vi "Arm Controller.vi"(8 "error in":errorcluster) -> ()   [LabVIEW 2023]
doc: "This VI executes continuously carrying out the current operation and responding to updates or new operations. It will often contain the timing or control code that is difficult to place directly in TeleOp. This VI generally opens all sensors and motors and isolates the rest of the robot code from knowing how the operations are carried out."
uses:
  <vilib>/Rock Robotics/WPI/Framework/Completion Status.ctl
  Arm Setpoints.ctl
  <vilib>/robotics/Kinematics/DH Dynamic Parameters.ctl
  <vilib>/Analysis/Matrix/Datatypes/RealMatrix.ctl
  <vilib>/robotics/Kinematics/DH Kinematic Parameters.ctl
  <vilib>/robotics/Kinematics/Link/Joint Type.ctl
  <vilib>/Rock Robotics/WPI/ThirdParty/REV Robotics/REVLib/Typedef/Spark MAX Control Type.ctl
  <vilib>/Rock Robotics/WPI/Solenoid/WPI_SolenoidValue.ctl
  <vilib>/robotics/Kinematics/Analytical/Initialize Generic Serial Arm.vi
  Framework/Robot Global Data.vi
  <vilib>/Rock Robotics/WPI/Solenoid/WPI_SolenoidSetEnum.vi
  <vilib>/robotics/Kinematics/Robot/Forward Kinematics (Point).vi
  <vilib>/robotics/Kinematics/Generate Cartesian Trajectory (Int).vi
  <vilib>/robotics/Kinematics/Robot/Inverse Kinematics (Point).vi
  <vilib>/robotics/Kinematics/Analytical/NI_Robotics_AnalyticKinematics.lvlib
  <vilib>/Analysis/Matrix/NI_Matrix.lvlib
  <vilib>/robotics/Kinematics/Link/NI_Robotics_Link.lvclass
  <vilib>/robotics/Kinematics/NI_Kinematics.lvlib
  <vilib>/robotics/Kinematics/Robot/NI_Robotics_Serial Robot Arm.lvclass
  <vilib>/Rock Robotics/Network Tables/NT Write Boolean.vi
panel:
  out "Output Lower":dbl
  out "Output Upper":dbl
  out "Sensor Position 4":dbl=277.41477272727275
  out "Sensor Position 3":dbl=225.42613636363637
  out "Applied Output 4":dbl
  out "Applied Output 3":dbl
  out "Applied Output 2":dbl
  in  "Arbitrary Feed Forward (0)":dbl=-0.1
  out "Applied Output":dbl
  out "Sensor Position 6":dbl=331.10795454545456
  out "Sensor Position 5":dbl=278.26704545454544
  in  "PID upper":T1={"P Gain"=0.8, "I Gain"=0.0, "D Gain"=0.0, "F Gain"=0.0, "I Zone"=0.0, "Min Output"=-1.0, "Max Output"=1.0}
  in  "PID Lower":T1={"P Gain"=2.0, "I Gain"=0.0, "D Gain"=0.0, "F Gain"=0.0, "I Zone"=0.0, "Min Output"=-1.0, "Max Output"=1.0}
  out "Sensor Position 2":dbl=187.5
  out "Sensor Position":dbl=124.00568181818183
  out "error out":errorcluster
  in  "Interactive Values":T2
  out "Current\nCmd":string="Started at  12:05:12.296\nDefault: Reserve,  S 0.0, D 0.000000"
  in  "Buttons":cluster{"Execute Cmd":bool, "Abort Cmd":bool}
  out "Command Timing":cluster{"Start Time (ms)":u32, "Iterations":i32}={"Start Time (ms)"=1211869, "Iterations"=0}
  out "Status":T3
  # "Tip: It may be helpful to observe inputs and sensor values.\nYou may also want to display tuning or debugging controls."
  # "Click here to set max"
  # "Click here to set min"
  # "Interactive Command: You may fill in the settings for a command\nand schedule it with the Execute button. You can observe and abort\nany command while fine tuning the code for the controller."
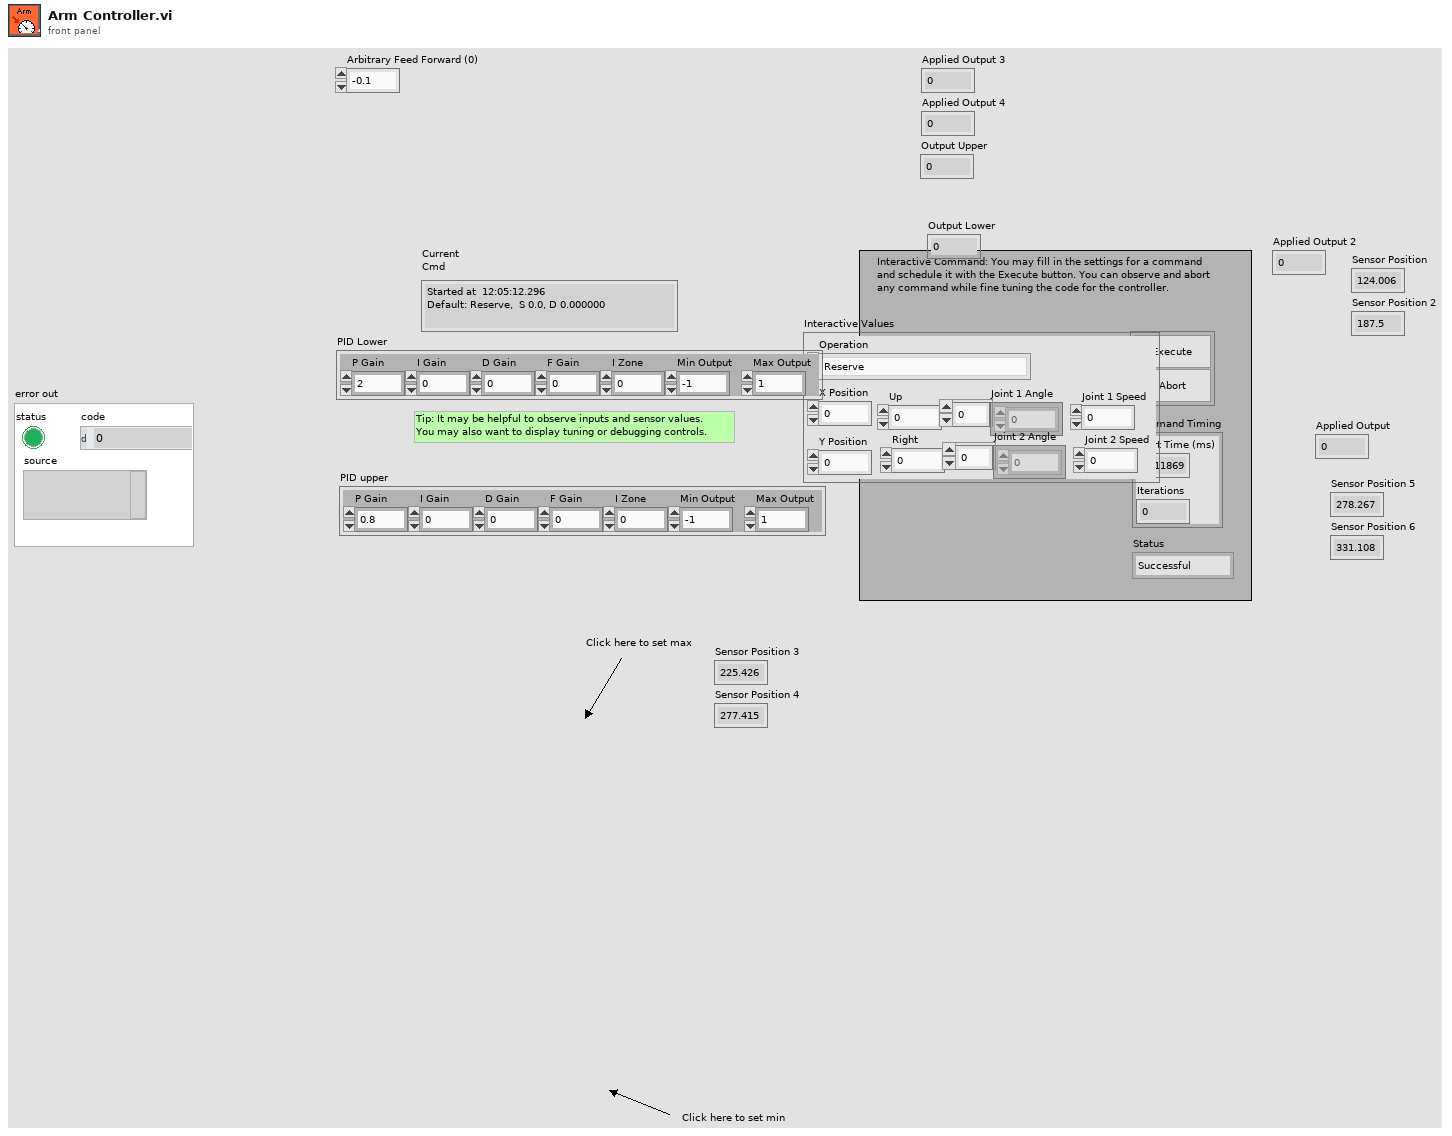
[diagram p1: front panel]
types:
  T1 = cluster{"P Gain":dbl, "I Gain":dbl, "D Gain":dbl, "F Gain":dbl, "I Zone":dbl, "Min Output":dbl, "Max Output":dbl}
  T2 = typedef "Arm Setpoints.ctl" = cluster{"Operation":enum16{"Reserve", "Read Current", "Immediate", "Move to position", "Adjust position", "Cube extend", "Cone extend", "Rotate Arm Joints", "Maintain Angle", "Retract", "Go_to_next"}, "X Position":dbl, "Y Position":dbl, "Up":dbl, "Right":dbl, "Joint 1 Angle":dbl[], "Joint 2 Angle":dbl[], "Joint 1 Speed":dbl, "Joint 2 Speed":dbl}
  T3 = typedef "Completion Status.ctl" = enum16{"Successful", "Aborted", "Incomplete"}
  T4 = typedef "DH Kinematic Parameters.ctl" = cluster{"twist angle":dbl, "length":dbl, "rotation angle":dbl, "offset distance":dbl, "joint type":T5, "joint coordinate offset":dbl}
  T5 = typedef "NI_Robotics_Link.lvclass/Joint Type.ctl" = enum16{"Revolute", "Prismatic"}
  T6 = typedef "DH Dynamic Parameters.ctl" = cluster{"mass":dbl, "gear ratio":dbl, "motor inertia":dbl, "center of gravity":dbl[], "viscous friction":dbl, "positive coulomb friction":dbl, "negative coulomb friction":dbl, "inertia matrix":T7}
  T7 = typedef "NI_Matrix.lvlib/RealMatrix.ctl" = dbl[][]
  T8 = typedef "Command Status Info.ctl" = cluster{"Name":string, "Status":T3, "notifier out":T9}
  T9 = typedef "Completion Notifier.ctl" = refnum<notifier>
  T10 = cluster{"Current Command":T2, "Command Timing":cluster{"Start Time (ms)":u32, "Iterations":i32}, "Command Arguments":cluster{"Command Info":T8, "Description":string, "Default Command":T2, "queue out":refnum<queue>, "Subsystem Name":string}}
  T11 = typedef "Spark MAX Control Type.ctl" = enum16{"Percent VBus", "Voltage", "Velocity", "Position", "Smart Motion", "Current", "Smart Velocity"}
  T12 = typedef "WPI_SolenoidValue.ctl" = enum16{"Off", "On", "Forward", "Reverse"}
  T13 = enum16{"Reserve", "Read Current", "Immediate", "Move to position", "Adjust position", "Cube extend", "Cone extend", "Rotate Arm Joints", "Maintain Angle", "Retract", "Go_to_next"}
  T14 = typedef "WPI_MotorControlDeviceRef.ctl" = cluster{"DeviceStatus":errorcluster, "Type":T15, "PWM":cluster{"PWM Channel":T16, "DeadBand":T17}, "CAN":cluster{"Device Number":u8, "SetOutput VI Ref":variant, "GetOutput VI Ref":variant, "Enable VI Ref":variant, "Disable VI Ref":variant, "Data":variant}, "Invert":bool, "DIO PWM":cluster{"PWM \"Enable\" Channel":T16, "DIOChannel":T18, "PWM Rate":dbl}}
  T15 = typedef "WPI_MotorControlType.ctl" = enum16{"PWM", "CAN", "DIO PWM"}
  T16 = typedef "FPGA_DIOPWMChannel.ctl" = enum8{"PWM 0", "PWM 1", "PWM 2", "PWM 3", "PWM 4", "PWM 5", "PWM 6", "PWM 7", "PWM 8", "PWM 9", "PWM MXP 0", "PWM MXP 1", "PWM MXP 2", "PWM MXP 3", "PWM MXP 4", "PWM MXP 5", "PWM MXP 6", "PWM MXP 7", "PWM MXP 8", "PWM MXP 9", "Invalid"}
  T17 = typedef "WPI_PWMDeadband.ctl" = cluster{"Name":string, "maxPositivePwm":i32, "minPositivePwm":i32, "centerPwm":i32, "maxNegativePwm":i32, "minNegativePwm":i32, "angularRange":u16}
  T18 = typedef "FPGA_DIOChannel.ctl" = enum8{"DIO 0", "DIO 1", "DIO 2", "DIO 3", "DIO 4", "DIO 5", "DIO 6", "DIO 7", "DIO 8", "DIO 9", "DIO MXP 0", "DIO MXP 1", "DIO MXP 2", "DIO MXP 3", "DIO MXP 4", "DIO MXP 5", "DIO MXP 6", "DIO MXP 7", "DIO MXP 8", "DIO MXP 9", "DIO MXP 10", "DIO MXP 11", "DIO MXP 12", "DIO MXP 13", "DIO MXP 14", "DIO MXP 15", "SPI Port CS1", "SPI Port CS2", "SPI Port CS3", "SPI Port MISO", "SPI Port MOSI", "Invalid"}
  T19 = typedef "WPI_SolenoidDevRef.ctl" = cluster{"DevStatus":errorcluster, "Pneumatics Control Module":u8, "Forward Solenoid Channel":T20, "Reverse Solenoid Channel":T20}
  T20 = typedef "WPI_SolenoidChannel.ctl" = enum8{"Solenoid 0", "Solenoid 1", "Solenoid 2", "Solenoid 3", "Solenoid 4", "Solenoid 5", "Solenoid 6", "Solenoid 7", "Solenoid 8", "Solenoid 9", "Solenoid 10", "Solenoid 11", "Solenoid 12", "Solenoid 13", "Solenoid 14", "Solenoid 15", "Invalid"}
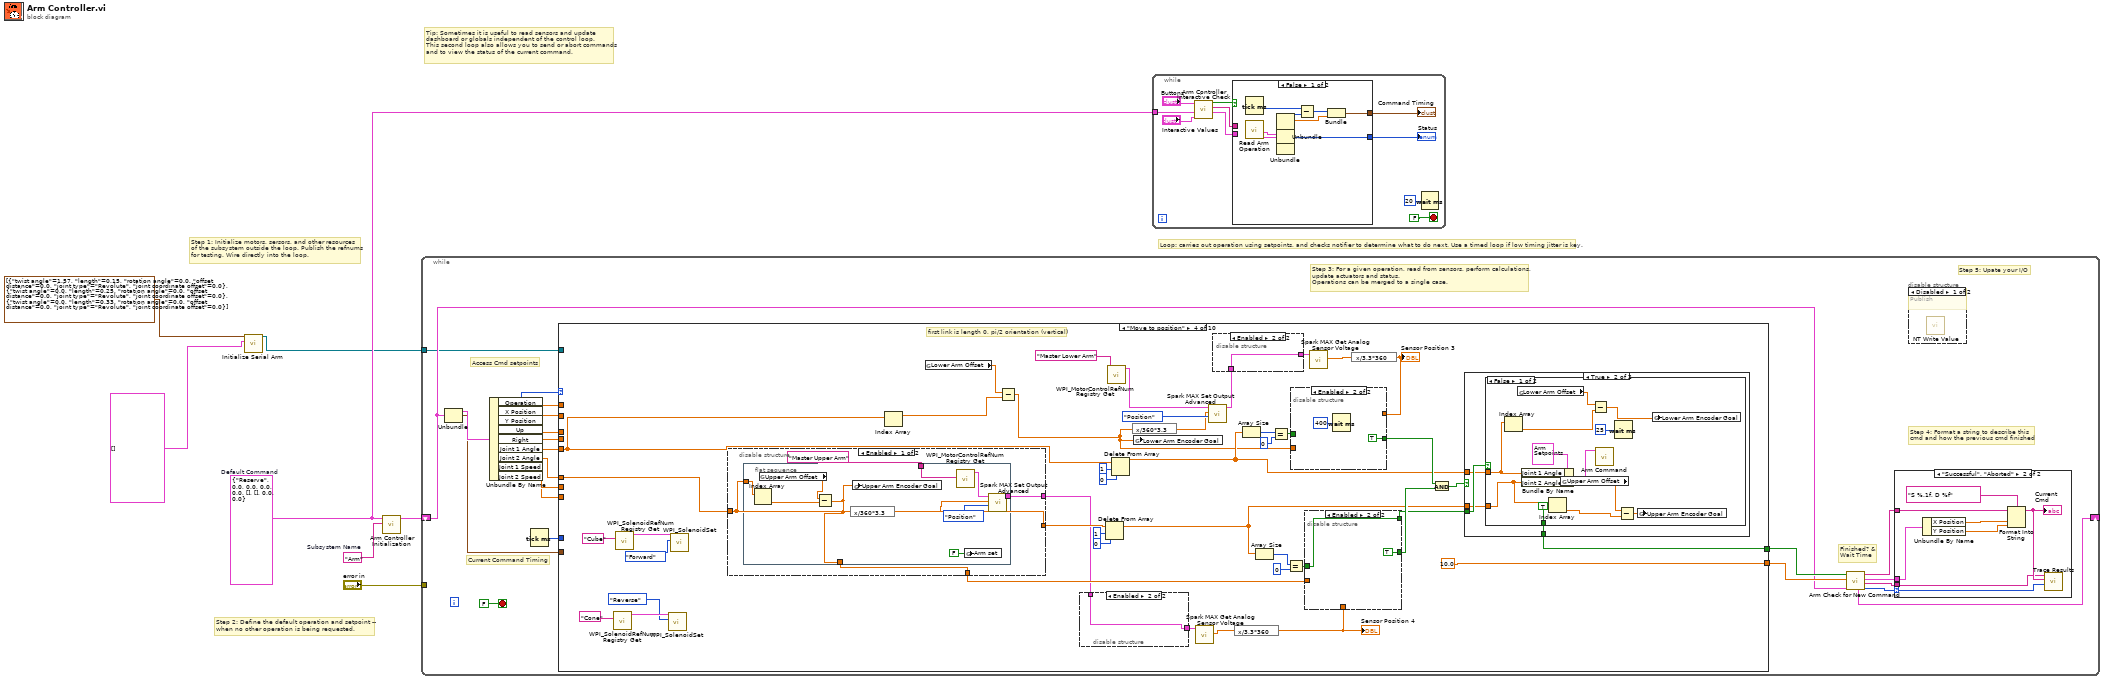
[diagram p0: block diagram]
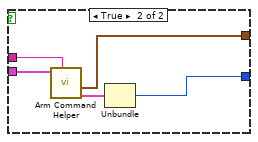
[diagram p2: hidden frame]
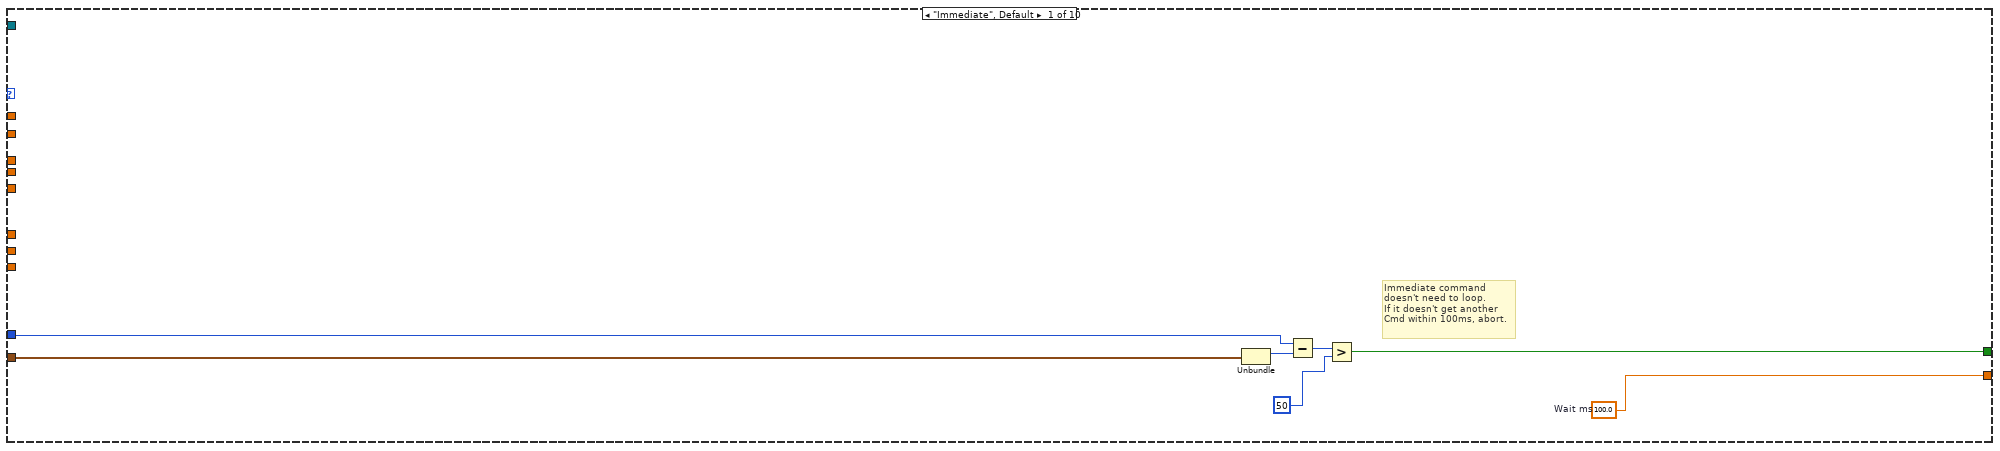
[diagram p3: hidden frame]
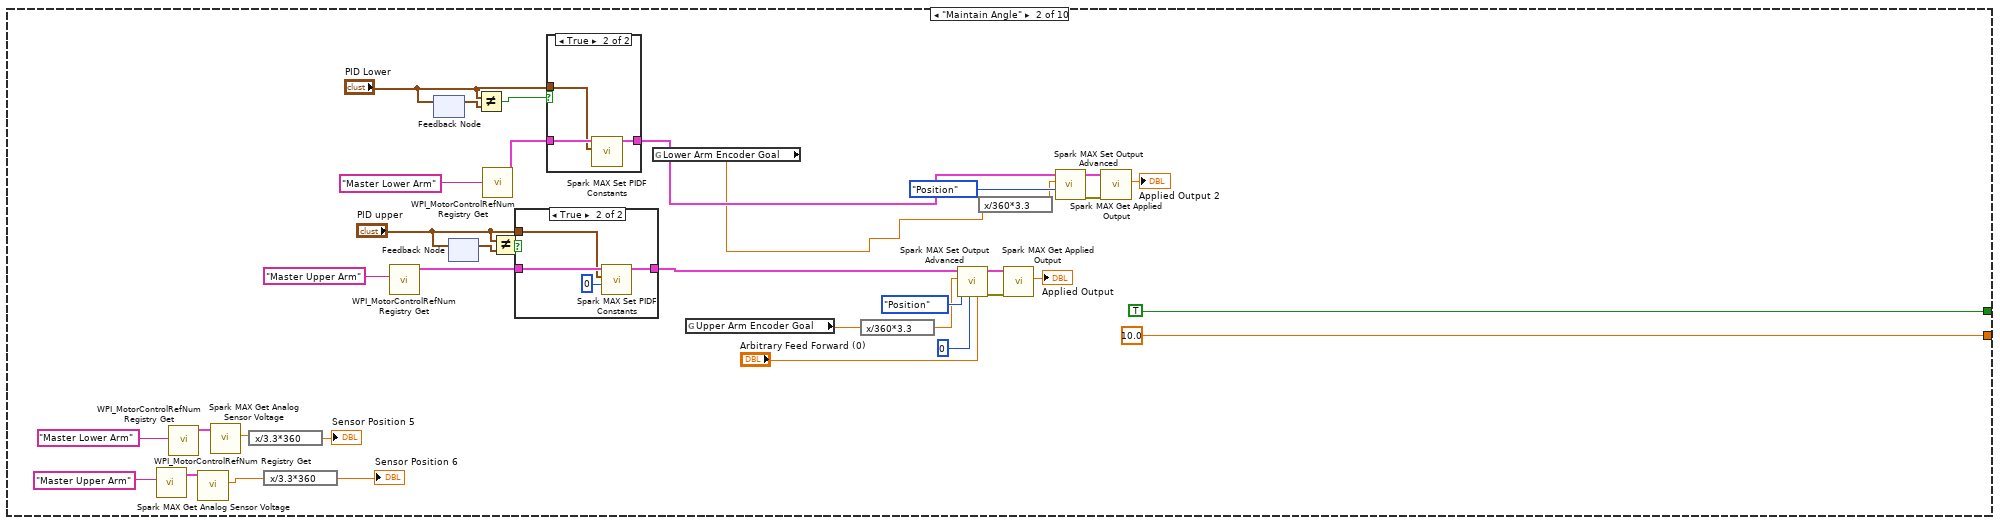
[diagram p4: hidden frame]
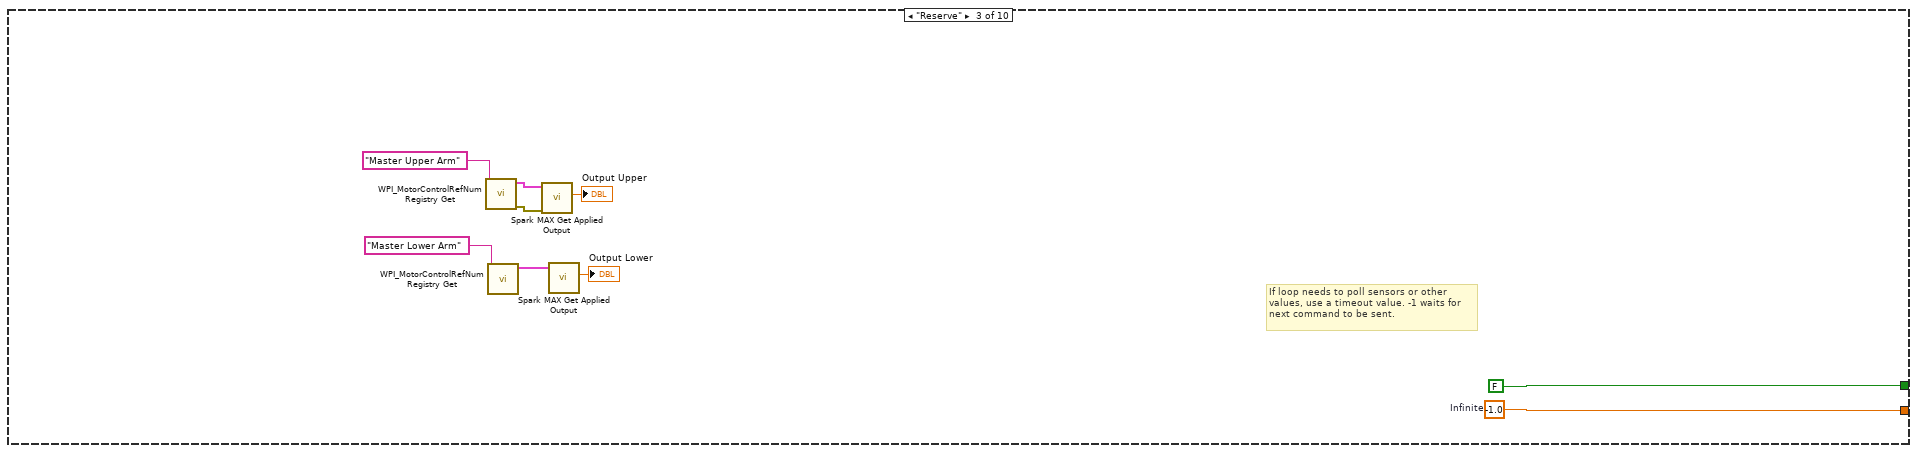
[diagram p7: hidden frame]
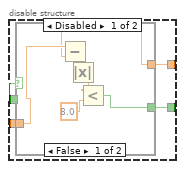
[diagram p8: hidden frame]
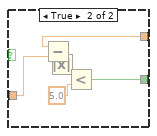
[diagram p9: hidden frame]
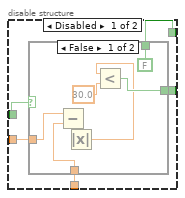
[diagram p10: hidden frame]
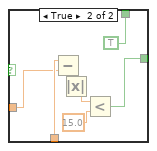
[diagram p11: hidden frame]
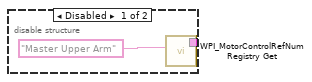
[diagram p12: hidden frame]
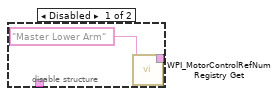
[diagram p13: hidden frame]
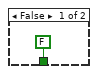
[diagram p14: hidden frame]
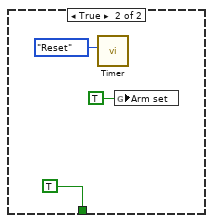
[diagram p15: hidden frame]
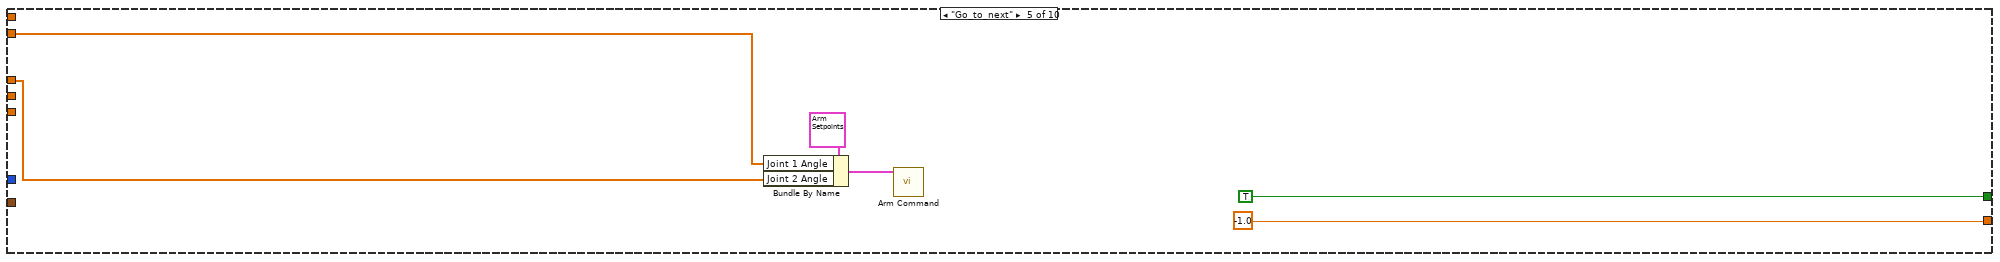
[diagram p17: hidden frame]
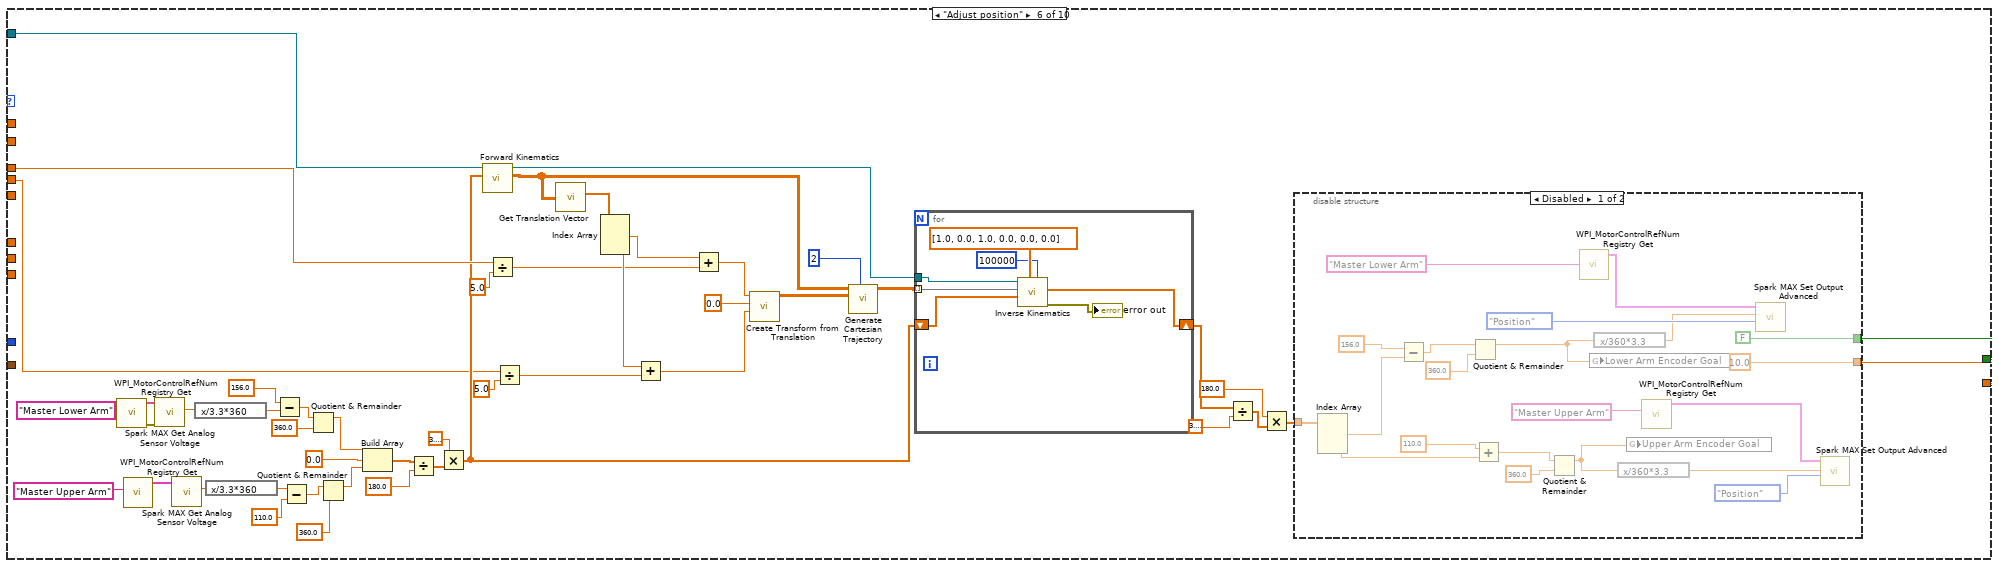
[diagram p18: hidden frame]
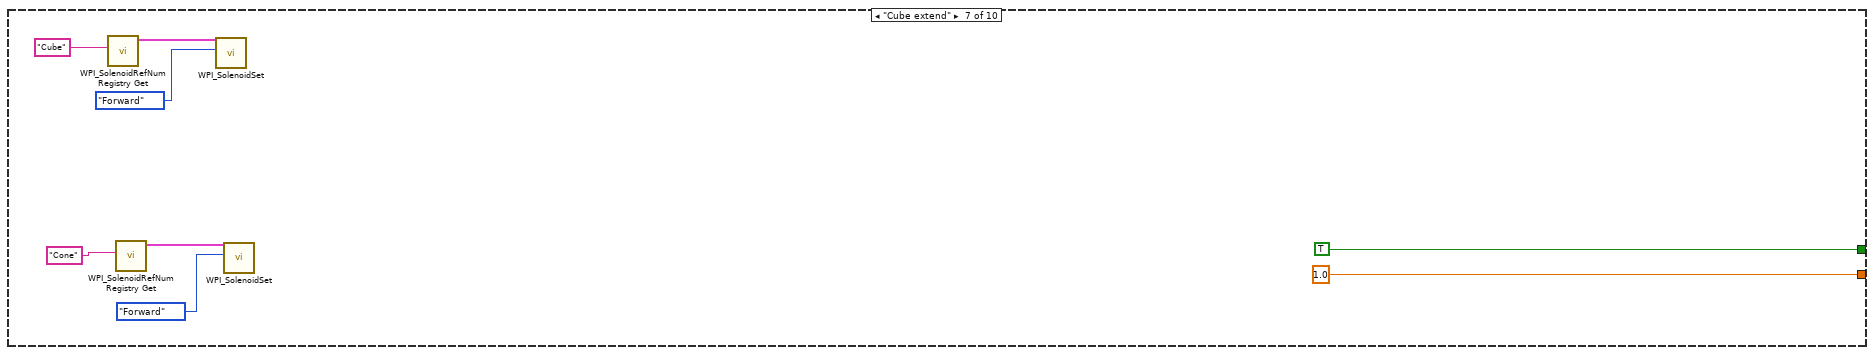
[diagram p20: hidden frame]
diagram:
  w4 = T2 {"Operation"=enum."Reserve", "X Position"=0.0, "Y Position"=0.0, "Up"=0.0, "Right"=0.0, "Joint 1 Angle"=[], "Joint 2 Angle"=[], "Joint 1 Speed"=0.0, "Joint 2 Speed"=0.0}  # Default Command
  w5 = "Arm"  # Subsystem Name
  # "Tip: Sometimes it is useful to read sensors and update\ndashboard or globals independent of the control loop.\nThis second loop also allows you to send or abort commands\nand to view the status of the current command."
  # "Step 2: Define the default operation and setpoint --\nwhen no other operation is being requested."
  # "Step 1: Initialize motors, sersors, and other resources\nof the subsystem outside the loop. Publish the refnums\nfor testing. Wire directly into the loop."
  # "Loop: carries out operation using setpoints, and checks notifier to determine what to do next. Use a timed loop if low timing jitter is key."
  n1 = call-poly <vilib>:"Initialize Serial Arm.vi"("dynamic parameters"=T6[] [], "kinematic parameters"=T4[] [{"twist angle"=1.57, "length"=0.15, "rotation angle"=0.0, "offset distance"=0.0, "joint type"=enum."Revolute", "joint coordinate offset"=0.0}, {"twist angle"=0.0, "length"=0.25, "rotation angle"=0.0, "offset distance"=0.0, "joint type"=enum."Revolute", "joint coordinate offset"=0.0}, {"twist angle"=0.0, "length"=0.33, "rotation angle"=0.0, "offset distance"=0.0, "joint type"=enum."Revolute", "joint coordinate offset"=0.0}]) -> ("serial arm out"=w1:refnum<class "NI_Robotics_Serial Robot Arm.lvclass">)  [unwired: 8 in, 1 out]
  n2 = call "Arm Controller Initialization.vi"("Subsystem Name"=w5, "Default Command"=w4) -> ("Current Command"=w6:T10)  [unwired: 9 in]
  n3 = while {
    shift-right: [w22] -> _
    shift-left: w6 -> [w15]
    tunnel: "error in" -> [_]
    tunnel: w1 -> [w14]
    stop <- FALSE stop-if-true
    # "Step 5: Upate your I/O"
    # "Step 4: Format a string to describe this\ncmd and how the previous cmd finished"
    # "Current Command Timing"
    # "Access Cmd setpoints"
    # "Finished? &\nWait Time"
    # "Step 3: For a given operation, read from sensors, perform calculations,\nupdate actuators and status.\nOperations can be merged to a single case."
    n4 = Unbundle(w15) -> ("Current Command"=w28:T2, "Command Timing"=w24:cluster{"Start Time (ms)":u32, "Iterations":i32})  [unwired: 1 out]
    n5 = Unbundle By Name(w28) -> ("Operation"=w27:T13, "X Position"=w26:dbl, "Y Position"=w23:dbl, "Up"=w13:dbl, "Right"=w12:dbl, "Joint 1 Angle"=w11:dbl[], "Joint 2 Angle"=w10:dbl[], "Joint 1 Speed"=w9:dbl, "Joint 2 Speed"=w8:dbl)
    n6 = Tick Count (ms)() -> (millisecond timer value=w25:u32)
    n7 = case shown="\"Move to position\"" w27 {
      tunnel: [w36 10.0 ("Infinite") w90 10.0 ("Infinite") -1.0 ("Infinite") w250 1.0 ("Infinite") 1.0 ("Infinite") 1.0 ("Infinite") 100.0 ("Infinite")] -> w20
      tunnel: [w30 TRUE ("ignore previous (F)") FALSE ("ignore previous (F)") w112 TRUE ("ignore previous (F)") w251 TRUE ("ignore previous (F)") TRUE ("ignore previous (F)") TRUE ("ignore previous (F)") TRUE ("ignore previous (F)")] -> w21
      tunnel: w24 -> [w32 _ _ _ _ _ _ _ _ _]
      tunnel: w26 -> [_ _ _ _ _ _ _ _ _ _]
      tunnel: w25 -> [w31 _ _ _ _ _ _ _ _ _]
      tunnel: w23 -> [_ _ _ _ _ _ _ _ _ _]
      tunnel: w14 -> [_ _ _ _ _ w258 _ _ _ _]
      tunnel: w13 -> [_ _ _ _ _ w252 _ _ _ _]
      tunnel: w12 -> [_ _ _ _ _ w236 _ _ _ _]
      tunnel: w11 -> [_ _ _ w102 w216 _ _ _ _ _]
      tunnel: w10 -> [_ _ _ w103 w215 _ _ _ _ _]
      tunnel: w9 -> [_ _ _ _ _ _ _ _ _ w341]
      tunnel: w8 -> [_ _ _ _ _ _ _ _ _ w340]
      frame "Immediate", Default {
        w36 = 100.0  # Wait ms
        # "Immediate command\ndoesn't need to loop.\nIf it doesn't get another\nCmd within 100ms, abort."
        n8 = Unbundle(w32) -> ("Start Time (ms)"=w35:u32)  [unwired: 1 out]
        n9 = Subtract(x=w31, y=w35) -> (x-y=w34:u32)
        n10 = Greater?(x=w34, y=u8 50 ("Left Motor")) -> (0:w30:bool)
      }
      frame "Maintain Angle" {
        n11 = call <vilib>:"WPI_MotorControlRefNum Registry Get.vi"("refnum name"="Master Upper Arm") -> ("MotorControlDevRef"=w59:T14)  [unwired: 9 in, 1 out]
        n12 = call <vilib>:"WPI_MotorControlRefNum Registry Get.vi"("refnum name"="Master Lower Arm") -> ("MotorControlDevRef"=w60:T14)  [unwired: 9 in, 1 out]
        n13 = call <vilib>:"Spark MAX Get Analog Sensor Voltage.vi"("MotorControlDevRef in"=w59) -> ("Analog Sensor Voltage"=w58:dbl)  [unwired: 7 in, 3 out]
        n14 = call <vilib>:"Spark MAX Get Analog Sensor Voltage.vi"("MotorControlDevRef in"=w60) -> ("Analog Sensor Voltage"=w57:dbl)  [unwired: 7 in, 3 out]
        n15 = expression code="x/3.3*360"(w57) -> (→"Sensor Position 5":dbl)
        n16 = expression code="x/3.3*360"(w58) -> (→"Sensor Position 6":dbl)
        n17 = call <vilib>:"WPI_MotorControlRefNum Registry Get.vi"("refnum name"="Master Upper Arm") -> ("MotorControlDevRef"=w69:T14)  [unwired: 9 in, 1 out]
        n18 = feedback #1() -> (w53:T1)  [unwired: 1 in]
        n19 = feedback-in #1("PID Lower") -> ()
        n20 = feedback-in #2("PID upper") -> ()
        n21 = feedback #2() -> (w55:T1)  [unwired: 1 in]
        n22 = Not Equal?(x="PID Lower", y=w53) -> (x != y?=w52:bool)
        n23 = call <vilib>:"WPI_MotorControlRefNum Registry Get.vi"("refnum name"="Master Lower Arm") -> ("MotorControlDevRef"=w71:T14)  [unwired: 9 in, 1 out]
        n24 = Not Equal?(x="PID upper", y=w55) -> (x != y?=w54:bool)
        n25 = case shown="True" w54 {
          tunnel: w69 -> [w77 w81]
          tunnel: "PID upper" -> [_ w80]
          tunnel: [w77 w79] -> w67
          frame False {
          }
          frame True {
            n26 = call <vilib>:"Spark MAX Set PIDF Constants.vi"("PIDF Slot"=0, "PID Constants"=w80, "MotorControlDeviceRef"=w81) -> ("MotorControlDeviceRef"=w79:T14)  [unwired: 7 in, 1 out]
          }
        }
        n27 = case shown="True" w52 {
          tunnel: w71 -> [w73 w76]
          tunnel: [w73 w75] -> w68
          tunnel: "PID Lower" -> [_ w74]
          frame False {
          }
          frame True {
            n28 = call <vilib>:"Spark MAX Set PIDF Constants.vi"("PID Constants"=w74, "MotorControlDeviceRef"=w76) -> ("MotorControlDeviceRef"=w75:T14)  [unwired: 8 in, 1 out]
          }
        }
        n29 = global read "Robot Global Data.vi" "Lower Arm Encoder Goal"() -> (w38:dbl)
        n30 = global read "Robot Global Data.vi" "Upper Arm Encoder Goal"() -> (w37:dbl)
        n31 = expression code="x/360*3.3"(w37) -> (w44:dbl)
        n32 = call <vilib>:"Spark MAX Set Output Advanced.vi"("Arbitrary Feed Forward (0)"="Arbitrary Feed Forward (0)", "PIDF Slot (0)"=0, "Control Mode"=Spark_MAX_Control_Type."Position", "Setpoint"=w44, "MotorControlDevRef"=w67) -> ("error out"=w49:errorcluster, "MotorControlDevRef"=w48:T14)  [unwired: 5 in]
        n33 = expression code="x/360*3.3"(w38) -> (w42:dbl)
        n34 = call <vilib>:"Spark MAX Get Applied Output.vi"("error in (no error)"=w49, "MotorControlDevRef in"=w48) -> ("Applied Output"=→"Applied Output":dbl)  [unwired: 6 in, 3 out]
        n35 = call <vilib>:"Spark MAX Set Output Advanced.vi"("Control Mode"=Spark_MAX_Control_Type."Position", "Setpoint"=w42, "MotorControlDevRef"=w68) -> ("error out"=w39:errorcluster, "MotorControlDevRef"=w40:T14)  [unwired: 7 in]
        n36 = call <vilib>:"Spark MAX Get Applied Output.vi"("error in (no error)"=w39, "MotorControlDevRef in"=w40) -> ("Applied Output"=→"Applied Output 2":dbl)  [unwired: 6 in, 3 out]
      }
      frame "Reserve" {
        w90 = -1.0  # Infinite
        # "If loop needs to poll sensors or other\nvalues, use a timeout value. -1 waits for\nnext command to be sent."
        n37 = call <vilib>:"WPI_MotorControlRefNum Registry Get.vi"("refnum name"="Master Upper Arm") -> ("error out"=w86:errorcluster, "MotorControlDevRef"=w85:T14)  [unwired: 9 in]
        n38 = call <vilib>:"WPI_MotorControlRefNum Registry Get.vi"("refnum name"="Master Lower Arm") -> ("MotorControlDevRef"=w82:T14)  [unwired: 9 in, 1 out]
        n39 = call <vilib>:"Spark MAX Get Applied Output.vi"("error in (no error)"=w86, "MotorControlDevRef in"=w85) -> ("Applied Output"=→"Output Upper":dbl)  [unwired: 6 in, 3 out]
        n40 = call <vilib>:"Spark MAX Get Applied Output.vi"("MotorControlDevRef in"=w82) -> ("Applied Output"=→"Output Lower":dbl)  [unwired: 7 in, 3 out]
      }
      frame "Move to position" {
        # "first link is length 0, pi/2 orientation (vertical)"
        n41 = call <vilib>:"WPI_SolenoidRefNum Registry Get.vi"("refnum name"="Cone") -> ("SolenoidDevRef"=w106:T19)  [unwired: 9 in, 1 out]
        n42 = call <vilib>:"WPI_SolenoidRefNum Registry Get.vi"("refnum name"="Cube") -> ("SolenoidDevRef"=w109:T19)  [unwired: 9 in, 1 out]
        n43 = call-poly <vilib>:"WPI_SolenoidSet.vi"("Value"=WPI_SolenoidValue."Reverse", "SolenoidDevRef"=w106) -> ()  [unwired: 8 in, 2 out]
        n44 = call-poly <vilib>:"WPI_SolenoidSet.vi"("Value"=WPI_SolenoidValue."Forward", "SolenoidDevRef"=w109) -> ()  [unwired: 8 in, 2 out]
        n45 = disable-structure shown="Enabled" {
          disable-tunnel: w103 -> [w201 _]
          disable-tunnel: [w201 _] -> w125
          disable-tunnel: [w200 _] -> w115
          disable-tunnel: [w199 _] -> w97
          frame Enabled {
            n46 = flat-sequence {
              tunnel: "Master Upper Arm" ("refnum name") -> [w210]
              tunnel: w201 -> [w209]
              tunnel: [w205] -> w200
              tunnel: [w206] -> w199
              frame #0 {
                n47 = Index Array(array=w209) -> (element=w203:dbl)  [unwired: 1 in]
                n48 = global read "Robot Global Data.vi" "Upper Arm Offset"() -> (w204:dbl)
                n49 = Subtract(x=w204, y=w203) -> (x-y=w205:dbl)
                n50 = expression code="x/360*3.3"(w205) -> (w208:dbl)
                n51 = global write "Robot Global Data.vi" "Upper Arm Encoder Goal"(w205) -> ()
                n52 = call <vilib>:"WPI_MotorControlRefNum Registry Get.vi"("refnum name"=w210) -> ("MotorControlDevRef"=w211:T14)  [unwired: 9 in, 1 out]
                n53 = global write "Robot Global Data.vi" "Arm set"(FALSE ("Arm set")) -> ()
                n54 = call <vilib>:"Spark MAX Set Output Advanced.vi"("Control Mode"=Spark_MAX_Control_Type."Position", "Setpoint"=w208, "MotorControlDevRef"=w211) -> ("MotorControlDevRef"=w206:T14)  [unwired: 7 in, 1 out]
              }
            }
          }
          frame Disabled {
          }
        }
        n55 = Index Array(array=w102) -> (element=w91:dbl)  [unwired: 1 in]
        n56 = global read "Robot Global Data.vi" "Lower Arm Offset"() -> (w92:dbl)
        n57 = Subtract(x=w92, y=w91) -> (x-y=w93:dbl)
        n58 = disable-structure shown="Enabled" {
          disable-tunnel: [w173 w175] -> w119
          disable-tunnel: w97 -> [_ w175]
          frame Disabled {
            n59 = call <vilib>:"WPI_MotorControlRefNum Registry Get.vi"("refnum name"="Master Upper Arm") -> ("MotorControlDevRef"=w173:T14)  [unwired: 9 in, 1 out]
          }
          frame Enabled {
          }
        }
        n60 = Delete From Array(array=w125, length=1, index=0) -> (array with subset deleted=w110:dbl[])  [unwired: 1 out]
        n61 = call <vilib>:"WPI_MotorControlRefNum Registry Get.vi"("refnum name"="Master Lower Arm") -> ("MotorControlDevRef"=w130:T14)  [unwired: 9 in, 1 out]
        n62 = Delete From Array(array=w102, length=1, index=0) -> (array with subset deleted=w111:dbl[])  [unwired: 1 out]
        n63 = expression code="x/360*3.3"(w93) -> (w101:dbl)
        n64 = global write "Robot Global Data.vi" "Lower Arm Encoder Goal"(w93) -> ()
        n65 = call <vilib>:"Spark MAX Get Analog Sensor Voltage.vi"("MotorControlDevRef in"=w119) -> ("Analog Sensor Voltage"=w118:dbl)  [unwired: 7 in, 3 out]
        n66 = call <vilib>:"Spark MAX Set Output Advanced.vi"("Control Mode"=Spark_MAX_Control_Type."Position", "Setpoint"=w101, "MotorControlDevRef"=w130) -> ("MotorControlDevRef"=w98:T14)  [unwired: 7 in, 1 out]
        n67 = disable-structure shown="Enabled" {
          disable-tunnel: [w176 w178] -> w120
          disable-tunnel: w98 -> [_ w178]
          frame Disabled {
            n68 = call <vilib>:"WPI_MotorControlRefNum Registry Get.vi"("refnum name"="Master Lower Arm") -> ("MotorControlDevRef"=w176:T14)  [unwired: 9 in, 1 out]
          }
          frame Enabled {
          }
        }
        n69 = expression code="x/3.3*360"(w118) -> (w99:dbl)
        "Sensor Position 4" <- w99
        n70 = Array Size(array=w111) -> (size(s)=w122:i32)
        n71 = Array Size(array=w110) -> (size(s)=w95:i32)
        n72 = Equal?(x=w122, y=0) -> (x = y?=w123:bool)
        n73 = Equal?(x=w95, y=0) -> (x = y?=w96:bool)
        n74 = disable-structure shown="Enabled" {
          disable-tunnel: w115 -> [w156 _]
          disable-tunnel: [w155 TRUE] -> w114
          disable-tunnel: [w154 w171] -> w113
          disable-tunnel: w99 -> [w153 _]
          disable-tunnel: w96 -> [w152 w171]
          frame Disabled {
            n75 = case shown="False" w152 {
              tunnel: w156 -> [w159 w164]
              tunnel: [w162 w169] -> w155
              tunnel: [FALSE TRUE] -> w154
              tunnel: w153 -> [w158 w166]
              frame False {
                n76 = Subtract(x=w159, y=w158) -> (x-y=w160:dbl)
                n77 = Absolute Value(x=w160) -> (abs(x)=w157:dbl)
                n78 = Less?(x=w157, y=30.0) -> (x < y?=w162:bool)
              }
              frame True {
                n79 = Subtract(x=w166, y=w164) -> (x-y=w167:dbl)
                n80 = Absolute Value(x=w167) -> (abs(x)=w165:dbl)
                n81 = Less?(x=w165, y=15.0) -> (x < y?=w169:bool)
              }
            }
          }
          frame Enabled {
          }
        }
        n82 = call <vilib>:"Spark MAX Get Analog Sensor Voltage.vi"("MotorControlDevRef in"=w120) -> ("Analog Sensor Voltage"=w117:dbl)  [unwired: 7 in, 3 out]
        n83 = expression code="x/3.3*360"(w117) -> (w100:dbl)
        "Sensor Position 3" <- w100
        n84 = disable-structure shown="Enabled" {
          disable-tunnel: w123 -> [w137 _]
          disable-tunnel: [w136 TRUE] -> w116
          disable-tunnel: w93 -> [w135 _]
          disable-tunnel: w100 -> [w134 _]
          frame Disabled {
            n85 = case shown="False" w137 {
              tunnel: [w142 w149] -> w136
              tunnel: w135 -> [w139 w146]
              tunnel: w134 -> [w138 w144]
              frame False {
                n86 = Subtract(x=w139, y=w138) -> (x-y=w141:dbl)
                n87 = Absolute Value(x=w141) -> (abs(x)=w140:dbl)
                n88 = Less?(x=w140, y=8.0) -> (x < y?=w142:bool)
              }
              frame True {
                n89 = Subtract(x=w144, y=w146) -> (x-y=w147:dbl)
                n90 = Absolute Value(x=w147) -> (abs(x)=w145:dbl)
                n91 = Less?(x=w145, y=5.0) -> (x < y?=w149:bool)
              }
            }
          }
          frame Enabled {
            n92 = Wait (ms)(milliseconds to wait=u32 400) -> ()  [unwired: 1 out]
          }
        }
        n93 = And(x=w116, y=w114) -> (x .and. y?=w121:bool)
        n94 = case shown="True" w121 {
          tunnel: w113 -> [_ w183]
          tunnel: [FALSE w182] -> w112
          tunnel: w111 -> [_ w181]
          tunnel: w110 -> [_ w180]
          frame False {
          }
          frame True {
            n95 = case shown="False" w183 {
              tunnel: [TRUE TRUE] -> w182
              tunnel: w181 -> [w191 _]
              tunnel: w180 -> [w190 _]
              frame False {
                n96 = Index Array(array=w191) -> (element=w185:dbl)  [unwired: 1 in]
                n97 = global read "Robot Global Data.vi" "Lower Arm Offset"() -> (w186:dbl)
                n98 = Bundle By Name(cluster=T2 {"Operation"=enum."Move to position", "X Position"=0.0, "Y Position"=0.0, "Up"=0.0, "Right"=0.0, "Joint 1 Angle"=[], "Joint 2 Angle"=[], "Joint 1 Speed"=0.0, "Joint 2 Speed"=0.0} ("SubSystem Data"), "Joint 1 Angle"=w191, "Joint 2 Angle"=w190) -> (w193:T2)
                n99 = Index Array(array=w190) -> (element=w188:dbl)  [unwired: 1 in]
                n100 = global read "Robot Global Data.vi" "Upper Arm Offset"() -> (w189:dbl)
                n101 = Subtract(x=w186, y=w185) -> (x-y=w184:dbl)
                n102 = call "Arm Command.vi"("SubSystem Data"=w193) -> ()  [unwired: 10 in, 1 out]
                n103 = Wait (ms)(milliseconds to wait=u32 25 ("millisecond timer value")) -> ()  [unwired: 1 out]
                n104 = Subtract(x=w189, y=w188) -> (x-y=w187:dbl)
                n105 = global write "Robot Global Data.vi" "Upper Arm Encoder Goal"(w187) -> ()
                n106 = global write "Robot Global Data.vi" "Lower Arm Encoder Goal"(w184) -> ()
              }
              frame True {
                n107 = call "Timer.vi"("Action"=enum16{"Reset", "Get"}."Reset") -> ()  [unwired: 10 in, 1 out]
                n108 = global write "Robot Global Data.vi" "Arm set"(TRUE ("Arm set")) -> ()
              }
            }
          }
        }
      }
      frame "Go_to_next" {
        n109 = Bundle By Name(cluster=T2 {"Operation"=enum."Move to position", "X Position"=0.0, "Y Position"=0.0, "Up"=0.0, "Right"=0.0, "Joint 1 Angle"=[], "Joint 2 Angle"=[], "Joint 1 Speed"=0.0, "Joint 2 Speed"=0.0} ("SubSystem Data"), "Joint 1 Angle"=w216, "Joint 2 Angle"=w215) -> (w217:T2)
        n110 = call "Arm Command.vi"("SubSystem Data"=w217) -> ()  [unwired: 10 in, 1 out]
      }
      frame "Adjust position" {
        n111 = call <vilib>:"WPI_MotorControlRefNum Registry Get.vi"("refnum name"="Master Lower Arm") -> ("error out"=w232:errorcluster, "MotorControlDevRef"=w233:T14)  [unwired: 9 in]
        n112 = call <vilib>:"WPI_MotorControlRefNum Registry Get.vi"("refnum name"="Master Upper Arm") -> ("MotorControlDevRef"=w230:T14)  [unwired: 9 in, 1 out]
        n113 = call <vilib>:"Spark MAX Get Analog Sensor Voltage.vi"("error in (no error)"=w232, "MotorControlDevRef in"=w233) -> ("Analog Sensor Voltage"=w231:dbl)  [unwired: 6 in, 3 out]
        n114 = call <vilib>:"Spark MAX Get Analog Sensor Voltage.vi"("MotorControlDevRef in"=w230) -> ("Analog Sensor Voltage"=w229:dbl)  [unwired: 7 in, 3 out]
        n115 = expression code="x/3.3*360"(w231) -> (w228:dbl)
        n116 = expression code="x/3.3*360"(w229) -> (w223:dbl)
        n117 = Subtract(x=156.0, y=w228) -> (x-y=w225:dbl)
        n118 = Subtract(x=w223, y=110.0) -> (x-y=w221:dbl)
        n119 = Quotient & Remainder(x=w225, y=360.0) -> (x-y*floor(x/y)=w226:dbl)  [unwired: 1 out]
        n120 = Quotient & Remainder(x=w221, y=360.0) -> (x-y*floor(x/y)=w219:dbl)  [unwired: 1 out]
        n121 = Build Array(w226, 0.0 ("element"), w219) -> (w247:dbl[])
        n122 = Divide(x=w247, y=180.0 ("x")) -> (x/y=w266:dbl[])
        n123 = Multiply(x=3.141592653589793, y=w266) -> (x*y=w245:dbl[])
        n124 = call-poly <vilib>:"Forward Kinematics.vi"("joint positions"=w245, "serial arm in"=w258) -> ("end effector transform"=w243:T7, "serial arm out"=w261:refnum<class "NI_Robotics_Serial Robot Arm.lvclass">)  [unwired: 7 in, 1 out]
        n125 = Divide(x=w252, y=5.0) -> (x/y=w238:dbl)
        n126 = Divide(x=w236, y=5.0) -> (x/y=w235:dbl)
        n127 = call <vilib>:"Get Translation Vector.vi"("transform"=w243) -> ("translation vector"=w242:dbl[])
        n128 = Index Array(array=w242) -> (element #1=w241:dbl, element #3=w240:dbl)  [unwired: 3 in, 1 out]
        n129 = Add(x=w240, y=w235) -> (x+y=w253:dbl)
        n130 = Add(x=w241, y=w238) -> (x+y=w244:dbl)
        n131 = call <vilib>:"Create Transform from Translation.vi"("z"=w253, "y"=0.0, "x"=w244) -> ("transform"=w262:T7)  [unwired: 8 in]
        n132 = call-poly <vilib>:"Generate Cartesian Trajectory.vi"("intermediate points"=2, "end transform"=w262, "start transform"=w243) -> ("interpolated trajectory"=w260:dbl[][][])  [unwired: 7 in, 1 out]
        n133 = for {
          tunnel: w261 -> [w294]
          tunnel: w260 -> [w293] mode=indexing
          shift-right: [w288] -> w254
          shift-left: w245 -> [w289]
          n134 = call-poly <vilib>:"Inverse Kinematics.vi"("max steps"=100000, "mask"=dbl[] [1.0, 0.0, 1.0, 0.0, 0.0, 0.0], "current joint positions"=w289, "end effector transform"=w293, "serial arm in"=w294) -> ("error out"=→"error out":errorcluster, "joint positions"=w288:dbl[])  [unwired: 3 in, 2 out]
        }
        n135 = Divide(x=w254, y=3.141592653589793) -> (x/y=w255:dbl[])
        n136 = Multiply(x=180.0, y=w255) -> (x*y=w248:dbl[])
        n137 = disable-structure shown="Disabled" {
          disable-tunnel: [FALSE ("ignore previous (F)") _] -> w251
          disable-tunnel: [10.0 ("Infinite") _] -> w250
          disable-tunnel: w248 -> [w285 _]
          frame Disabled {
            n138 = Index Array(array=w285) -> (element #1=w276:dbl, element #3=w273:dbl)  [unwired: 3 in, 1 out]
            n139 = Subtract(x=156.0, y=w276) -> (x-y=w271:dbl)
            n140 = Quotient & Remainder(x=w271, y=360.0) -> (x-y*floor(x/y)=w270:dbl)  [unwired: 1 out]
            n141 = Add(x=110.0, y=w273) -> (x+y=w268:dbl)
            n142 = Quotient & Remainder(x=w268, y=360.0) -> (x-y*floor(x/y)=w267:dbl)  [unwired: 1 out]
            n143 = call <vilib>:"WPI_MotorControlRefNum Registry Get.vi"("refnum name"="Master Lower Arm") -> ("MotorControlDevRef"=w279:T14)  [unwired: 9 in, 1 out]
            n144 = global write "Robot Global Data.vi" "Lower Arm Encoder Goal"(w270) -> ()
            n145 = expression code="x/360*3.3"(w270) -> (w281:dbl)
            n146 = expression code="x/360*3.3"(w267) -> (w283:dbl)
            n147 = global write "Robot Global Data.vi" "Upper Arm Encoder Goal"(w267) -> ()
            n148 = call <vilib>:"WPI_MotorControlRefNum Registry Get.vi"("refnum name"="Master Upper Arm") -> ("MotorControlDevRef"=w278:T14)  [unwired: 9 in, 1 out]
            n149 = call <vilib>:"Spark MAX Set Output Advanced.vi"("Control Mode"=Spark_MAX_Control_Type."Position", "Setpoint"=w281, "MotorControlDevRef"=w279) -> ()  [unwired: 7 in, 2 out]
            n150 = call <vilib>:"Spark MAX Set Output Advanced.vi"("Control Mode"=Spark_MAX_Control_Type."Position", "Setpoint"=w283, "MotorControlDevRef"=w278) -> ()  [unwired: 7 in, 2 out]
          }
          frame Enabled {
          }
        }
      }
      frame "Cube extend" {
        n151 = call <vilib>:"WPI_SolenoidRefNum Registry Get.vi"("refnum name"="Cube") -> ("SolenoidDevRef"=w302:T19)  [unwired: 9 in, 1 out]
        n152 = call <vilib>:"WPI_SolenoidRefNum Registry Get.vi"("refnum name"="Cone") -> ("SolenoidDevRef"=w297:T19)  [unwired: 9 in, 1 out]
        n153 = call-poly <vilib>:"WPI_SolenoidSet.vi"("Value"=WPI_SolenoidValue."Forward", "SolenoidDevRef"=w302) -> ()  [unwired: 8 in, 2 out]
        n154 = call-poly <vilib>:"WPI_SolenoidSet.vi"("Value"=WPI_SolenoidValue."Forward", "SolenoidDevRef"=w297) -> ()  [unwired: 8 in, 2 out]
      }
      frame "Cone extend" {
        n155 = flat-sequence {
          frame #0 {
            n156 = Wait (ms)(milliseconds to wait=u32 60 ("millisecond timer value")) -> ()  [unwired: 1 out]
          }
          frame #1 {
            n157 = call <vilib>:"WPI_SolenoidRefNum Registry Get.vi"("refnum name"="Cone") -> ("SolenoidDevRef"=w309:T19)  [unwired: 9 in, 1 out]
            n158 = call <vilib>:"WPI_SolenoidRefNum Registry Get.vi"("refnum name"="Cube") -> ("SolenoidDevRef"=w312:T19)  [unwired: 9 in, 1 out]
            n159 = call-poly <vilib>:"WPI_SolenoidSet.vi"("Value"=WPI_SolenoidValue."Reverse", "SolenoidDevRef"=w309) -> ()  [unwired: 8 in, 2 out]
            n160 = call-poly <vilib>:"WPI_SolenoidSet.vi"("Value"=WPI_SolenoidValue."Forward", "SolenoidDevRef"=w312) -> ()  [unwired: 8 in, 2 out]
            n161 = global write "Robot Global Data.vi" "Grabber State"(enum16{"Closed", "Open"}."Closed" ("Grabber State")) -> ()
          }
        }
      }
      frame "Retract" {
        n162 = call <vilib>:"WPI_SolenoidRefNum Registry Get.vi"("refnum name"="Cube") -> ("SolenoidDevRef"=w319:T19)  [unwired: 9 in, 1 out]
        n163 = call <vilib>:"WPI_SolenoidRefNum Registry Get.vi"("refnum name"="Cone") -> ("SolenoidDevRef"=w316:T19)  [unwired: 9 in, 1 out]
        n164 = call-poly <vilib>:"WPI_SolenoidSet.vi"("Value"=WPI_SolenoidValue."Reverse", "SolenoidDevRef"=w319) -> ()  [unwired: 8 in, 2 out]
        n165 = call-poly <vilib>:"WPI_SolenoidSet.vi"("Value"=WPI_SolenoidValue."Forward", "SolenoidDevRef"=w316) -> ()  [unwired: 8 in, 2 out]
        n166 = global write "Robot Global Data.vi" "Grabber State"(enum16{"Closed", "Open"}."Open" ("Grabber State")) -> ()
      }
      frame "Rotate Arm Joints" {
        w326 = 15.0 ("y")
        n167 = disable-structure shown="Enabled" {
          disable-tunnel: w341 -> [w359 w367]
          disable-tunnel: w340 -> [w354 w366]
          disable-tunnel: [_ w367] -> w339
          disable-tunnel: [_ w366] -> w338
          frame Disabled {
            w353 = 0.2 ("upper limit")
            w357 = 0.2 ("upper limit")
            n168 = call <vilib>:"WPI_MotorControlRefNum Registry Get.vi"("refnum name"="Master Upper Arm") -> ("MotorControlDevRef"=w362:T14)  [unwired: 9 in, 1 out]
            n169 = call <vilib>:"WPI_MotorControlRefNum Registry Get.vi"("refnum name"="Master Lower Arm") -> ("MotorControlDevRef"=w363:T14)  [unwired: 9 in, 1 out]
            n170 = Negate(x=w353) -> (-x=w355:dbl)
            n171 = Negate(x=w357) -> (-x=w356:dbl)
            n172 = In Range and Coerce(upper limit=w353, x=w354, lower limit=w355) -> (coerced(x)=w352:dbl)  [unwired: 1 out]
            n173 = In Range and Coerce(upper limit=w357, x=w359, lower limit=w356) -> (coerced(x)=w358:dbl)  [unwired: 1 out]
            n174 = call <vilib>:"Spark MAX Set Output Advanced.vi"("Control Mode"=Spark_MAX_Control_Type."Percent VBus", "Setpoint"=w352, "MotorControlDevRef"=w362) -> ()  [unwired: 7 in, 2 out]
            n175 = call <vilib>:"Spark MAX Set Output Advanced.vi"("Control Mode"=Spark_MAX_Control_Type."Percent VBus", "Setpoint"=w358, "MotorControlDevRef"=w363) -> ()  [unwired: 7 in, 2 out]
          }
          frame Enabled {
          }
        }
        n176 = call <vilib>:"WPI_MotorControlRefNum Registry Get.vi"("refnum name"="Master Upper Arm") -> ("MotorControlDevRef"=w346:T14)  [unwired: 9 in, 1 out]
        n177 = call <vilib>:"WPI_MotorControlRefNum Registry Get.vi"("refnum name"="Master Lower Arm") -> ("MotorControlDevRef"=w347:T14)  [unwired: 9 in, 1 out]
        n178 = call <vilib>:"Spark MAX Get Analog Sensor Voltage.vi"("MotorControlDevRef in"=w346) -> ("Analog Sensor Voltage"=w345:dbl, "MotorControlDevRef out"=w330:T14)  [unwired: 7 in, 2 out]
        n179 = call <vilib>:"Spark MAX Get Analog Sensor Voltage.vi"("MotorControlDevRef in"=w347) -> ("Analog Sensor Voltage"=w344:dbl, "MotorControlDevRef out"=w333:T14)  [unwired: 7 in, 2 out]
        n180 = expression code="x/3.3*360"(w344) -> (w343:dbl)
        "Sensor Position" <- w343
        n181 = expression code="x/3.3*360"(w345) -> (w342:dbl)
        "Sensor Position 2" <- w342
        n182 = Multiply(x=w326, y=w339) -> (x*y=w327:dbl)
        n183 = Multiply(x=w338, y=w326) -> (x*y=w328:dbl)
        n184 = Add(x=w327, y=w343) -> (x+y=w332:dbl)
        n185 = Add(x=w342, y=w328) -> (x+y=w331:dbl)
        n186 = global write "Robot Global Data.vi" "Lower Arm Encoder Goal"(w332) -> ()
        n187 = global write "Robot Global Data.vi" "Upper Arm Encoder Goal"(w331) -> ()
        n188 = expression code="x/360*3.3"(w332) -> (w334:dbl)
        n189 = expression code="x/360*3.3"(w331) -> (w336:dbl)
        n190 = call <vilib>:"Spark MAX Set Output Advanced.vi"("Control Mode"=Spark_MAX_Control_Type."Position", "Setpoint"=w334, "MotorControlDevRef"=w333) -> ("MotorControlDevRef"=w325:T14)  [unwired: 7 in, 1 out]
        n191 = call <vilib>:"Spark MAX Set Output Advanced.vi"("Control Mode"=Spark_MAX_Control_Type."Position", "Setpoint"=w336, "MotorControlDevRef"=w330) -> ("MotorControlDevRef"=w324:T14)  [unwired: 7 in, 1 out]
        n192 = call <vilib>:"Spark MAX Get Applied Output.vi"("MotorControlDevRef in"=w325) -> ("Applied Output"=→"Applied Output 4":dbl)  [unwired: 7 in, 3 out]
        n193 = call <vilib>:"Spark MAX Get Applied Output.vi"("MotorControlDevRef in"=w324) -> ("Applied Output"=→"Applied Output 3":dbl)  [unwired: 7 in, 3 out]
        n194 = Wait (ms)(milliseconds to wait=u32 100) -> ()  [unwired: 1 out]
      }
    }
    n195 = call "Arm Check for New Command.vi"("Current Command"=w15, "Wait time (ms)"=w20, "Finished?"=w21) -> ("Completion"=w16:T3, "Subsystem Name"=w17:string, "Current Command"=w18:T2, "Initial Trace String"=w19:string, "NextCommand"=w22:T10)  [unwired: 4 in]
    n196 = case shown="\"Successful\", \"Aborted\"" w16 {
      selector: w16 -> [_ w375]
      tunnel: w19 -> [_ w371]
      tunnel: w18 -> [_ w372]
      tunnel: w17 -> [_ w368]
      frame "Incomplete", Default {
        # "Continuing current command"
      }
      frame "Successful", "Aborted" {
        # "Report and setup for next command"
        n197 = Unbundle By Name(w372) -> ("X Position"=w374:dbl, "Y Position"=w369:dbl)
        n198 = Format Into String(format string="S %.1f, D %f", initial string=w371, w374, w369) -> (resulting string=w370:string)  [unwired: 1 in, 1 out]
        "Current\nCmd" <- w370
        n199 = call <vilib>:"Trace Results.vi"("Status of previous command"=w375, "Description"=w370, "Subsystem"=w368) -> ()  [unwired: 9 in]
      }
    }
    n200 = disable-structure shown="Disabled" {
      frame Disabled {
        # "Publish"
        n201 = call-poly <vilib>:"NT Write Value.vi"() -> ()  [unwired: 11 in, 1 out]
      }
      frame Enabled {
      }
    }
  }
  n202 = while {
    tunnel: w4 -> [w382]
    stop <- FALSE stop-if-true
    n203 = call "Arm Controller Interactive Check.vi"("Interactive Command in"="Interactive Values", "Default Command"=w382, "Buttons"="Buttons") -> ("Interactive Command out"=w379:T2, "Trace String"=w380:string, "Schedule"=w381:bool)  [unwired: 6 in]
    n204 = case shown="False" w381 {
      tunnel: [w393 w398] -> w378
      tunnel: w379 -> [_ w396]
      tunnel: [w389 w394] -> w377
      tunnel: w380 -> [_ w397]
      frame False {
        n205 = Tick Count (ms)() -> (millisecond timer value=w388:u32)
        n206 = call "Read Arm Operation.vi"() -> ("Command Info"=w386:T8, "SubSystem Data"=w387:T2)  [unwired: 9 in, 1 out]
        n207 = Unbundle(w387) -> ("Operation"=w392:T13, "X Position"=w390:dbl)  [unwired: 7 out]
        n208 = Unbundle(w386) -> ("Status"=w393:T3)  [unwired: 2 out]
        n209 = Subtract(x=w388, y=w392) -> (x-y=w391:u32)
        n210 = Bundle(w391, "X Position"=w390) -> (w389:cluster{u32, "X Position":dbl})  [unwired: 1 in]
      }
      frame True {
        n211 = call "Arm Command Helper.vi"("Description"=w397, "SubSystem Data"=w396) -> ("Command Info Out"=w395:T8, "Command Timing"=w394:cluster{"Start Time (ms)":u32, "Iterations":i32})  [unwired: 7 in, 1 out]
        n212 = Unbundle(w395) -> ("Status"=w398:T3)  [unwired: 2 out]
      }
    }
    "Status" <- w378
    "Command Timing" <- w377
    n213 = Wait (ms)(milliseconds to wait=u32 20) -> ()  [unwired: 1 out]
  }
